vi "calc_motors.vi"(7 "resonator_motor, f(x)":string, 8 "error in (no error)":errorcluster, 10 "wavelength (nm)":dbl format="%0.2f") -> (0 "error out":errorcluster, 2 "resonator":i32)   [LabVIEW 2017, in "sirah.lvlib"]
uses:
  sirah.lvlib
  <vilib>/gmath/NI_Gmath.lvlib
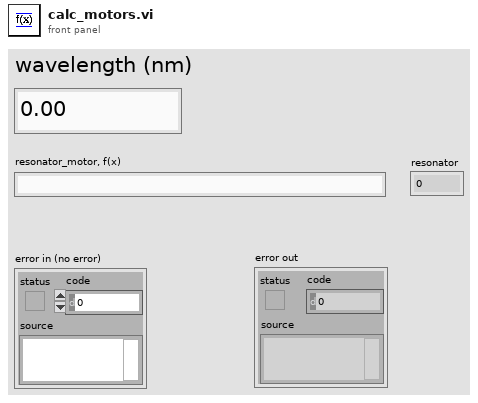
[diagram p1: front panel]
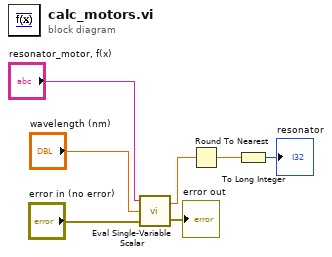
[diagram p0: block diagram]
diagram:
  n1 = call <vilib>:"Eval Single-Variable Scalar.vi"("error in (no error)"="error in (no error)", "x value"="wavelength (nm)", "formula"="resonator_motor, f(x)") -> ("error out"=→"error out":errorcluster, "y value"=w6:dbl)
  n2 = Round To Nearest(number=w6) -> (nearest integer value=w5:dbl)
  n3 = To Long Integer(number=w5) -> (32bit integer=→"resonator":i32)
